vi "CODCr通讯.vi"() -> ()   [LabVIEW 2016, in "CODCr库.lvlib"]
uses:
  <vilib>/Plasmionique/MB Master/MB_Master_TCP/MB_Master_TCP.lvclass
  D:/Program Files (x86)/National Instruments/LabVIEW 2016/vi.lib/Plasmionique/MB Master/MB_Master/MB_Master.lvclass
  <vilib>/NI/Modbus Library/API/Wrapper/Create TCP Slave.vi
  <vilib>/NI/Modbus Library/API/slave/Modbus Slave.lvclass
  <vilib>/Plasmionique/MB Master/MB Master.lvlib
  <vilib>/Utility/config.llb/NI_LVConfig.lvlib
  <vilib>/NI/Modbus Library/API/Wrapper/API Main.lvlib
  <vilib>/Plasmionique/MB Master/MB_Master/MB_Master.lvclass
panel:
  out "状态告警区":u16[](array[numeric])
  out "测量数据区":u16[](array[numeric])
  in  "读取参数":bool
  in  "读取数据":bool
  in  "释放串口":bool
  in  "打开串口":bool
  out "队列中元素数量":i32
  out "元素":cluster{"命令":string}[](array[cluster])
  out "待处理插入数量":i32
  out "读取公式":u16[](array[numeric])
  out "读取参数":u16[](array[numeric])
  out "数据存储":u16[](array[numeric])
  out "通讯状态":bool
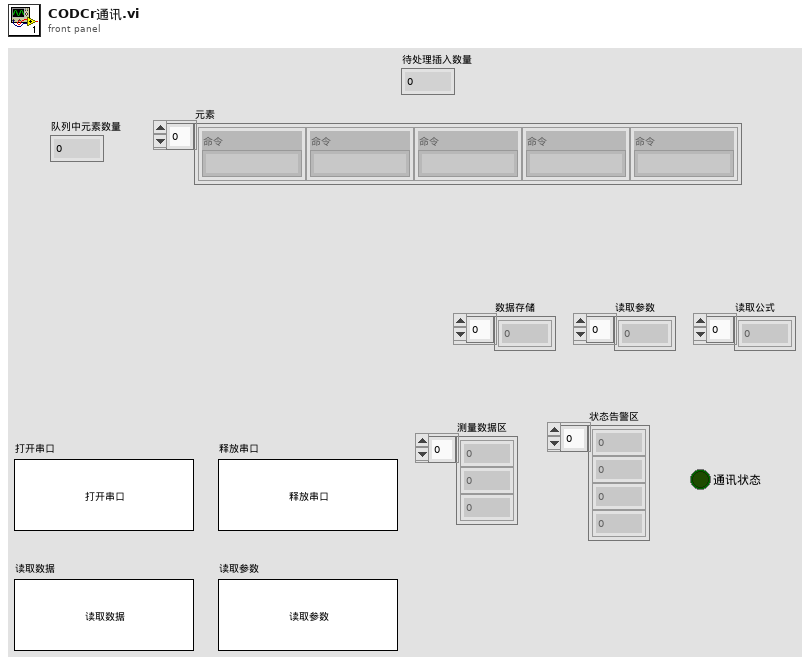
[diagram p1: front panel]
types:
  T1 = typedef "NI_LVConfig.lvlib/Config Data RefNum.ctl" = refnum<k1>
  T2 = cluster{"因子编码":u32, "单位":u16, "标样参考值":sgl, "水样数据时间":timestamp, "水样实测值":sgl, "水样数据标识":string, "标样数据时间":timestamp, "标样实测值":sgl, "标样数据标识":string, "空白数据时间":timestamp, "空白实测值":sgl, "空白数据标识":string, "零点核查数据时间":timestamp, "零点核查实测值":sgl, "零点核查数据标识":string, "跨度核查数据时间":timestamp, "跨度核查实测值":sgl, "跨度核查数据标识":string, "加标回收数据时间":timestamp, "加标回收实测值":sgl, "加标回收数据标识":string, "平行样数据时间":timestamp, "平行样实测值":sgl, "平行样数据标识":string}
  T3 = cluster{"系统时间":timestamp, "工作状态":enum16{"空闲", "水样测试", "标样核查", "零点核查", "跨度核查", "空白测试", "平行样测试", "加标回收", "空白校准", "标样校准", "初始化（清洗）"}, "测量模式":enum16{"待机", "连续模式", "周期模式", "定点模式", "受控模式", "手动模式"}, "告警代码":enum16{"无告警", "缺试剂告警", "缺水样告警", "缺蒸馏水告警", "缺标液告警", "仪表漏液告警", "标定异常告警", "超量程告警", "加热异常", "低试剂预警", "超上限告警", "超下限告警", "仪表内部其他异常", "滴定异常告警", "电极异常告警", "量程切换告警", "参数设置告警", "PH电极电位异常", "电导率电极异常", "浊度光度异常", "溶解氧电极异常", "溶解氧光强异常", "温度异常告警", "PH异常告警", "溶解氧异常告警", "电导率异常告警", "浊度异常告警", "叶绿素异常告警", "藻密度异常告警", "蓝绿藻异常告警", "ORP异常告警", "氨氮异常告警", "清洁刷异常告警", "SD卡异常告警", "蓝牙异常告警", "Wifi异常告警", "流程异常告警"}, "故障代码":enum16{"无故障", "电机故障", "温度故障", "通讯故障", "滴定故障"}, "日志代码":u16, "软件版本":u16, "F0":sgl, "F1":sgl, "F2":sgl, "F3":sgl, "T":sgl, "H":sgl, "id":u16, "flowid":u16, "量程":u16}
  T4 = cluster{"测量精度":u16, "消解温度":u16, "消解时长":u16, "量程下限":sgl, "量程上限":sgl, "曲线斜率K":sgl, "曲线斜率B":sgl, "标定日期":timestamp, "标液1浓度":sgl, "标液1测量过程值":sgl, "标液2浓度":sgl, "标液2测量过程值":sgl, "标液3浓度":sgl, "标液3测量过程值":sgl, "标液4浓度":sgl, "标液4测量过程值":sgl, "标液5浓度":sgl, "标液5测量过程值":sgl, "线性相关系数":sgl, "试剂余量":u32, "测量滴定值或吸光度":sgl, "空白校准时间":timestamp, "标样校准时间":timestamp, "检出限值":sgl, "校准系数":sgl, "设备系列号":string}
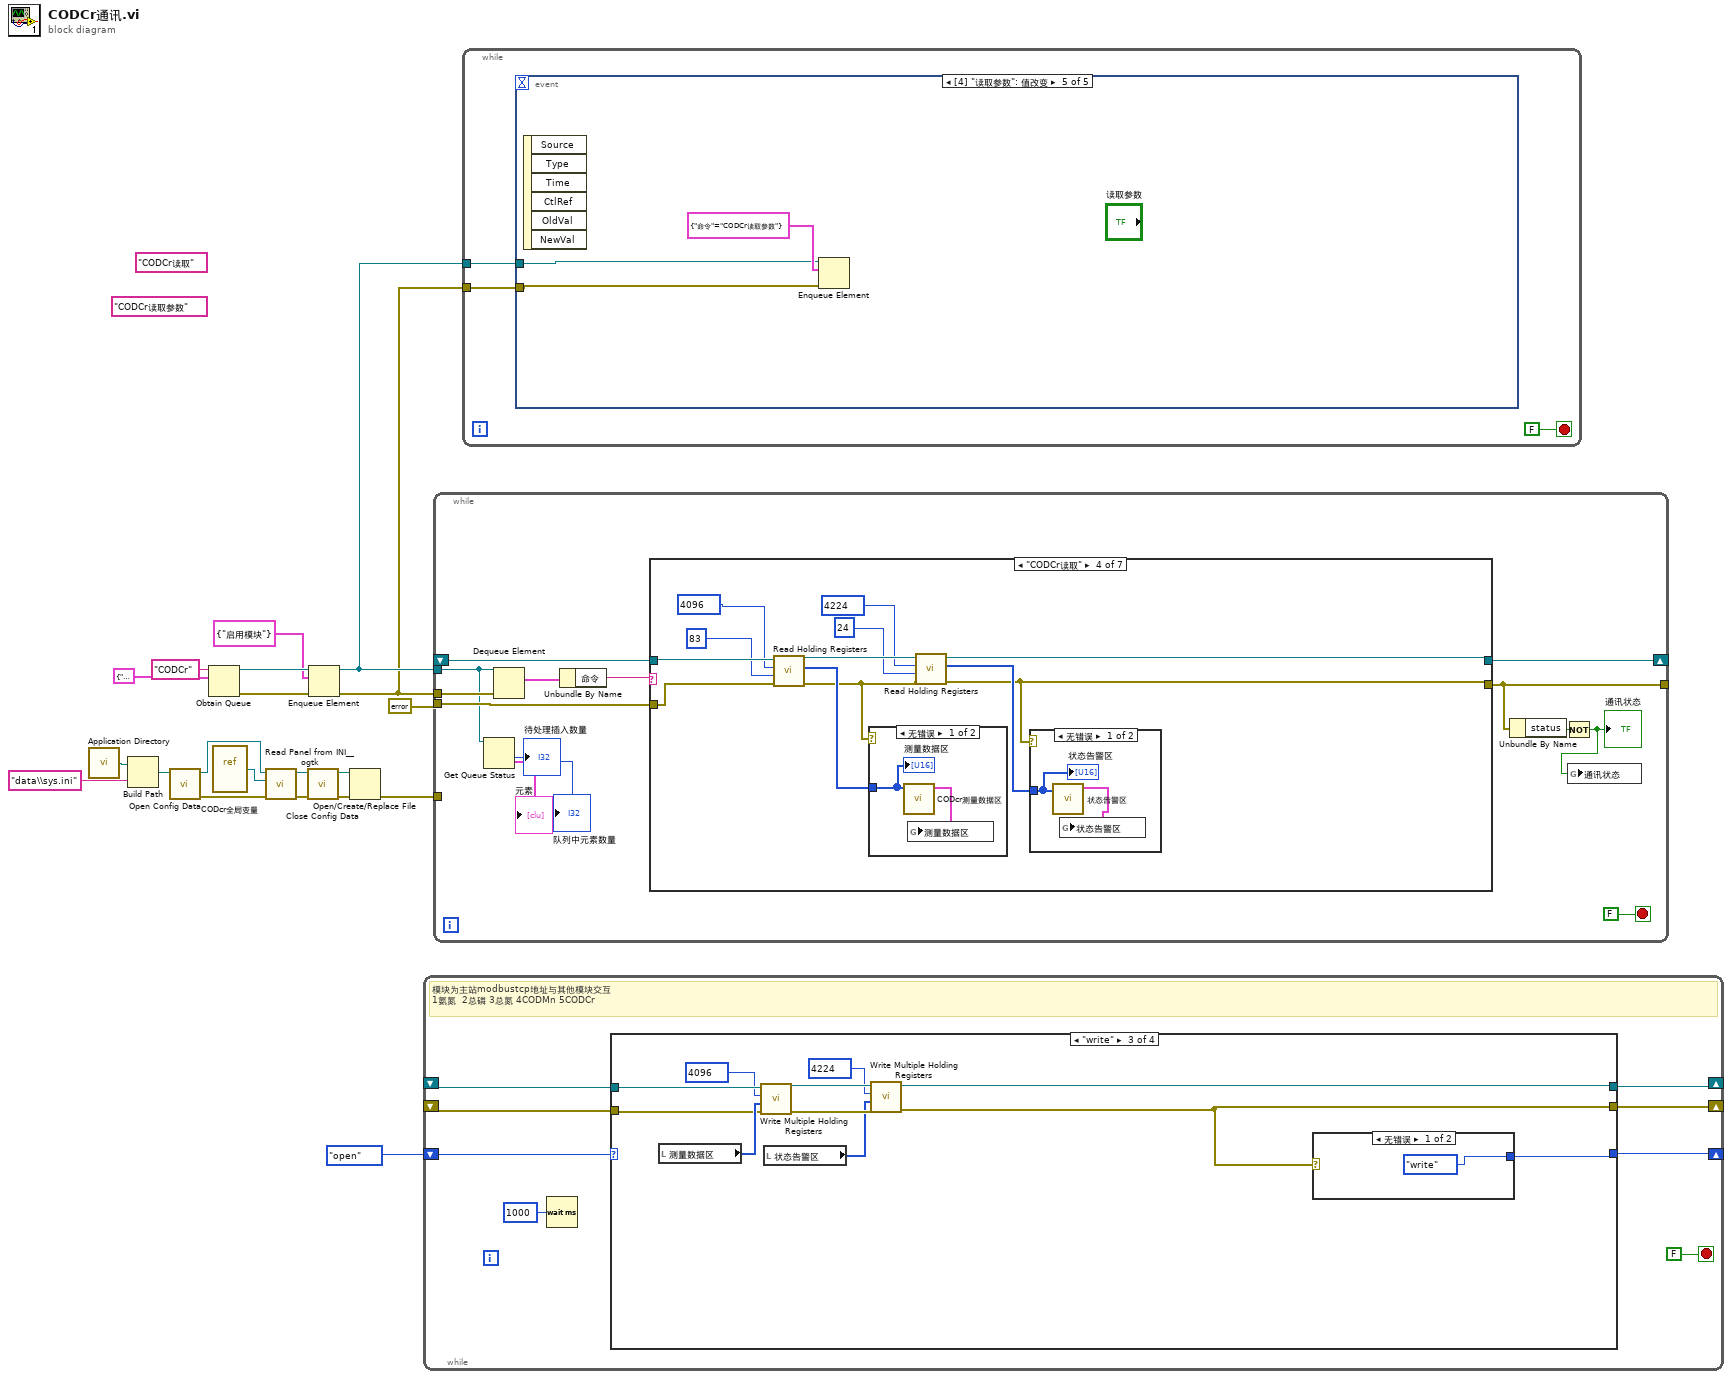
[diagram p0: block diagram]
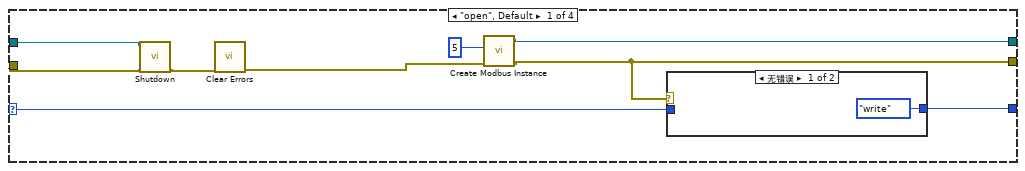
[diagram p2: hidden frame]
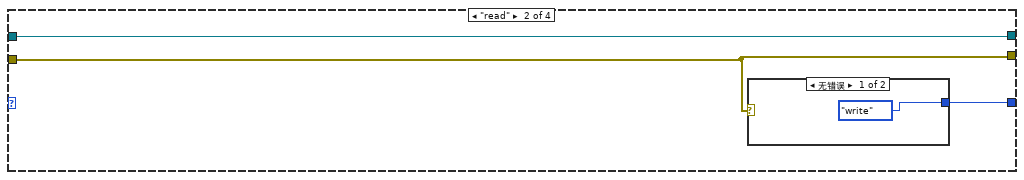
[diagram p4: hidden frame]
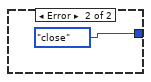
[diagram p5: hidden frame]
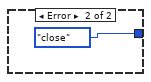
[diagram p6: hidden frame]
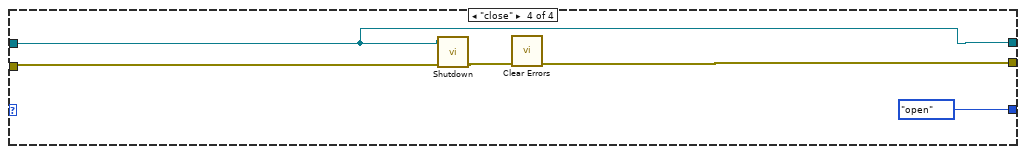
[diagram p7: hidden frame]
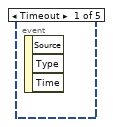
[diagram p8: hidden frame]
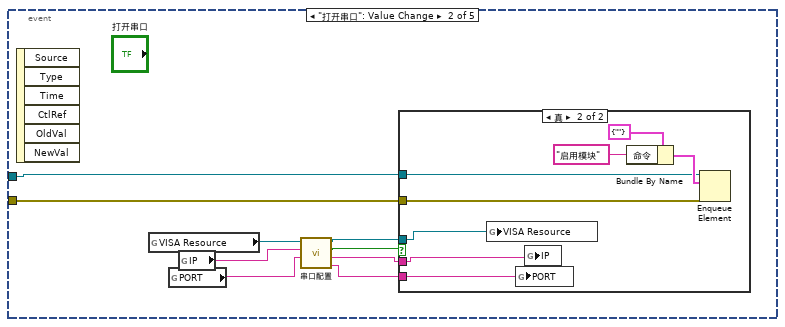
[diagram p9: hidden frame]
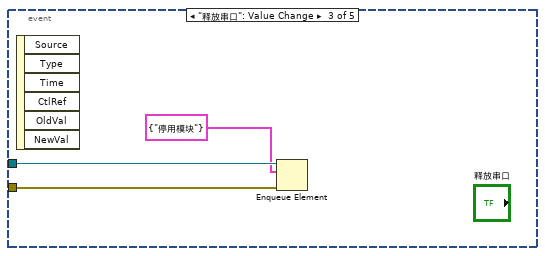
[diagram p11: hidden frame]
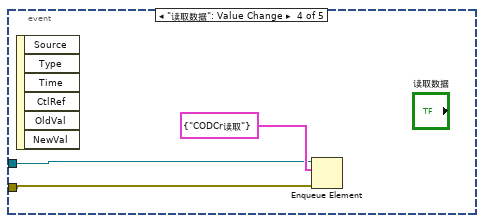
[diagram p12: hidden frame]
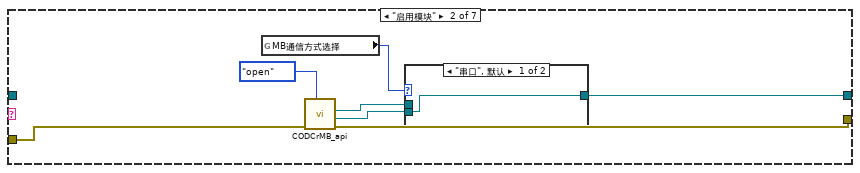
[diagram p14: hidden frame]
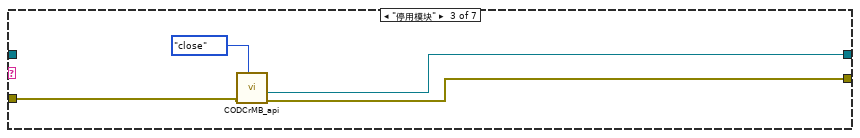
[diagram p16: hidden frame]
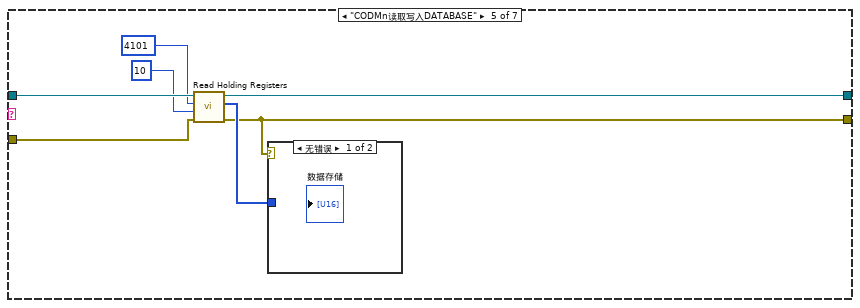
[diagram p19: hidden frame]
diagram:
  (unwired) "CODCr读取参数" ("名称（未命名）")
  (unwired) "CODCr读取" ("名称（未命名）")
  n1 = call <vilib>:"Application Directory.vi"() -> ("Application Directory"=w14:path)
  n2 = Build Path(base path=w14, name or relative path="data\\sys.ini" ("名称或相对路径")) -> (appended path=w12:path)
  n3 = call <vilib>:"Open Config Data.vi"("configuration file path"=w12) -> ("error out"=w8:errorcluster, "refnum"=w11:T1)  [unwired: 8 in, 1 out]
  n4 = Obtain Queue(name (unnamed)="CODCr" ("名称（未命名）"), element data type=cluster{"命令":string} {"命令"="启用模块"} ("元素")) -> (queue out=w17:refnum<queue>, error out=w16:errorcluster)  [unwired: 3 in, 1 out]
  n5 = vi-ref "CODcr全局变量.vi"() -> (w10:refnum<vi>)
  n6 = call <userlib>:"Read Panel from INI__ogtk.vi"("error in (no error)"=w8, "VI ref"=w10, "refnum"=w11) -> ("error out"=w7:errorcluster, "refnum out"=w9:T1)  [unwired: 7 in]
  n7 = call <vilib>:"Close Config Data.vi"("error in (no error)"=w7, "refnum"=w9) -> ("error out"=w6:errorcluster, "file path"=w5:path)  [unwired: 8 in]
  n8 = Enqueue Element(queue=w17, element=cluster{"命令":string} {"命令"="启用模块"} ("元素"), error in (no error)=w16) -> (queue out=w3:refnum<queue>, error out=w2:errorcluster)  [unwired: 1 in, 1 out]
  n9 = Open/Create/Replace File(file path (use dialog)=w5, error in=w6) -> (error out=w4:errorcluster)  [unwired: 4 in, 2 out]
  n10 = while {
    shift-right: [w26] -> _
    shift-left: _ -> [w28]
    shift-right: [w25] -> _
    shift-left: _ -> [w27]
    shift-right: [w22] -> _
    shift-left: enum16{"open", "read", "write", "close"}."open" -> [w23]
    stop <- FALSE stop-if-true
    # "模块为主站modbustcp地址与其他模块交互\n1氨氮  2总磷 3总氮 4CODMn 5CODCr"
    n11 = Wait (ms)(milliseconds to wait=u32 1000 ("等待时间（毫秒）")) -> ()  [unwired: 1 out]
    n12 = case shown="\"write\"" w23 {
      selector: w23 -> [w37 _ _ _]
      tunnel: w28 -> [w31 w40 w54 w60]
      tunnel: w27 -> [w30 w41 w50 w59]
      tunnel: [w34 w40 w46 w60] -> w26
      tunnel: [w33 w41 w45 w62] -> w25
      tunnel: [w36 w42 w55 enum16{"open", "read", "write", "close"}."open"] -> w22
      frame "open", Default {
        n13 = call-dynamic "Shutdown.vi"("error in"=w30, "Modbus slave in"=w31) -> ("error out"=w29:errorcluster)  [unwired: 9 in]
        n14 = call <vilib>:"Clear Errors.vi"("error in (no error)"=w29) -> ("error out"=w32:errorcluster)  [unwired: 5 in, 1 out]
        n15 = call-poly <vilib>:"Create Modbus Instance.vi"("error in"=w32, "port (502)"=u16 5) -> ("error out"=w33:errorcluster, "TCP slave instance"=w34:refnum<class "Modbus Slave.lvclass">)  [unwired: 8 in]
        n16 = case shown="无错误" w33 {
          tunnel: w37 -> [_ w39]
          tunnel: [enum16{"open", "read", "write", "close"}."write" w39] -> w36
          frame No Error {
          }
          frame Error {
          }
        }
      }
      frame "read" {
        n17 = case shown="无错误" w41 {
          tunnel: [enum16{"open", "read", "write", "close"}."write" enum16{"open", "read", "write", "close"}."close"] -> w42
          frame No Error {
          }
          frame Error {
          }
        }
      }
      frame "write" {
        n18 = local read "测量数据区"() -> (w52:u16[])
        n19 = call-dynamic "Write Multiple Holding Registers.vi"("error in"=w50, "registers to write"=w52, "starting address"=u16 4096, "Modbus slave in"=w54) -> ("error out"=w49:errorcluster, "Modbus slave out"=w51:refnum<class "Modbus Slave.lvclass">)  [unwired: 6 in]
        n20 = local read "状态告警区"() -> (w47:u16[])
        n21 = call-dynamic "Write Multiple Holding Registers.vi"("error in"=w49, "registers to write"=w47, "starting address"=u16 4224, "Modbus slave in"=w51) -> ("error out"=w45:errorcluster, "Modbus slave out"=w46:refnum<class "Modbus Slave.lvclass">)  [unwired: 6 in]
        n22 = case shown="无错误" w45 {
          tunnel: [enum16{"open", "read", "write", "close"}."write" enum16{"open", "read", "write", "close"}."close"] -> w55
          frame No Error {
          }
          frame Error {
          }
        }
      }
      frame "close" {
        n23 = call-dynamic "Shutdown.vi"("error in"=w59, "Modbus slave in"=w60) -> ("error out"=w58:errorcluster)  [unwired: 9 in]
        n24 = call <vilib>:"Clear Errors.vi"("error in (no error)"=w58) -> ("error out"=w62:errorcluster)  [unwired: 5 in, 1 out]
      }
    }
  }
  n25 = while {
    tunnel: w3 -> [w66]
    tunnel: w2 -> [w75]
    tunnel: [w67] -> _
    shift-right: [w71] -> _
    shift-left: _ -> [w70]
    tunnel: errorcluster {"status"=FALSE, "code"=0, "source"=""} ("error out") -> [w69]
    tunnel: w4 -> [_]
    stop <- FALSE stop-if-true
    n26 = Get Queue Status(queue=w66) -> (# pending insert=→"待处理插入数量":i32, # elements in queue=→"队列中元素数量":i32, elements=→"元素":cluster{"命令":string}[])  [unwired: 2 in, 5 out]
    n27 = Dequeue Element(queue=w66, error in (no error)=w75) -> (element=w74:cluster{"命令":string})  [unwired: 1 in, 3 out]
    n28 = Unbundle By Name(w74) -> ("命令"=w73:string)
    n29 = case shown="\"CODCr读取\"" w73 {
      tunnel: [w78 w79 w88 w97 w110 w118 w127] -> w71
      tunnel: [w77 w85 w89 w96 w108 w117 w126] -> w67
      tunnel: w70 -> [w78 _ _ w103 w114 w121 w130]
      tunnel: w69 -> [w77 w83 w90 w102 w111 w120 w129]
      frame Default {
      }
      frame "启用模块" {
        n30 = global read "CODcr全局变量.vi" "MB通信方式选择"() -> (w82:enum16{"串口", "TCP"})
        n31 = call "CODCrMB_api.vi"("STEP"=enum16{"open", "read", "write", "close"}."open", "Error in"=w83) -> ("error out"=w85:errorcluster, "MB session out"=w81:refnum<class "MB_Master.lvclass">, "MB_TCP session"=w80:refnum<class "MB_Master_TCP.lvclass">)  [unwired: 6 in, 1 out]
        n32 = case shown="\"串口\", 默认" w82 {
          tunnel: w81 -> [w86 _]
          tunnel: w80 -> [_ w87]
          tunnel: [w86 w87] -> w79
          frame "串口", Default {
          }
          frame "TCP" {
          }
        }
      }
      frame "停用模块" {
        n33 = call "CODCrMB_api.vi"("STEP"=enum16{"open", "read", "write", "close"}."close", "Error in"=w90) -> ("error out"=w89:errorcluster, "MB session out"=w88:refnum<class "MB_Master.lvclass">)  [unwired: 6 in, 2 out]
      }
      frame "CODCr读取" {
        n34 = call <vilib>:"Read Holding Registers.vi"("error in (no error)"=w102, "quantity"=u16 83 ("number of holding registers"), "starting address"=u16 4096, "MB session in"=w103) -> ("error out"=w99:errorcluster, "Registers"=w101:u16[], "MB session out"=w100:refnum<class "MB_Master.lvclass">)  [unwired: 5 in]
        n35 = case shown="无错误" w99 {
          tunnel: w101 -> [w106 _]
          frame No Error {
            n36 = call "CODcr测量数据区.vi"("数组"=w106) -> ("测量数据区"=w107:T2)  [unwired: 10 in]
            n37 = global write "CODcr全局变量.vi" "测量数据区"(w107) -> ()
            "测量数据区" <- w106
          }
          frame Error {
          }
        }
        n38 = call <vilib>:"Read Holding Registers.vi"("error in (no error)"=w99, "quantity"=u16 24 ("number of holding registers"), "starting address"=u16 4224, "MB session in"=w100) -> ("error out"=w96:errorcluster, "Registers"=w98:u16[], "MB session out"=w97:refnum<class "MB_Master.lvclass">)  [unwired: 5 in]
        n39 = case shown="无错误" w96 {
          tunnel: w98 -> [w104 _]
          frame No Error {
            n40 = call "状态告警区.vi"("数组"=w104) -> ("状态告警区"=w105:T3)  [unwired: 10 in]
            n41 = global write "CODcr全局变量.vi" "状态告警区"(w105) -> ()
            "状态告警区" <- w104
          }
          frame Error {
          }
        }
      }
      frame "CODMn读取写入DATABASE" {
        n42 = call <vilib>:"Read Holding Registers.vi"("error in (no error)"=w111, "quantity"=u16 10 ("number of holding registers"), "starting address"=u16 4101, "MB session in"=w114) -> ("error out"=w108:errorcluster, "Registers"=w109:u16[], "MB session out"=w110:refnum<class "MB_Master.lvclass">)  [unwired: 5 in]
        n43 = case shown="无错误" w108 {
          tunnel: w109 -> [_ _]
          frame No Error {
          }
          frame Error {
          }
        }
      }
      frame "CODCr读取参数" {
        n44 = call <vilib>:"Read Holding Registers.vi"("error in (no error)"=w120, "quantity"=u16 19 ("number of holding registers"), "starting address"=u16 4256, "MB session in"=w121) -> ("error out"=w117:errorcluster, "Registers"=w119:u16[], "MB session out"=w118:refnum<class "MB_Master.lvclass">)  [unwired: 5 in]
        n45 = case shown="无错误" w117 {
          tunnel: w119 -> [w122 _]
          frame No Error {
            n46 = call "关键参数区.vi"("数组"=w122) -> ("关键参数区"=w123:T4)  [unwired: 10 in]
            n47 = global write "CODcr全局变量.vi" "关键参数区"(w123) -> ()
          }
          frame Error {
          }
        }
      }
      frame "CODMn读取公式" {
        n48 = call <vilib>:"Read Holding Registers.vi"("error in (no error)"=w129, "quantity"=u16 94 ("number of holding registers"), "starting address"=u16 4616, "MB session in"=w130) -> ("error out"=w126:errorcluster, "Registers"=w128:u16[], "MB session out"=w127:refnum<class "MB_Master.lvclass">)  [unwired: 5 in]
        n49 = case shown="无错误" w126 {
          tunnel: w128 -> [_ _]
          frame No Error {
          }
          frame Error {
          }
        }
      }
    }
    n50 = Unbundle By Name(w67) -> ("status"=w72:bool)
    n51 = Not(x=w72) -> (.not. x?=w68:bool)
    "通讯状态" <- w68
    n52 = global write "CODcr全局变量.vi" "通讯状态"(w68) -> ()
  }
  n53 = while {
    tunnel: w3 -> [w132]
    tunnel: w2 -> [w131]
    stop <- FALSE stop-if-true
    n54 = event shown="[4] \"读取参数\": 值改变" {
      selector: _ -> [_ _ _ _ _]
      dyn-events: _ -> [_ _ _ _ _]
      timeout: _ -> [_ _ _ _ _]
      tunnel: w132 -> [_ w142 w153 w155 w158]
      tunnel: w131 -> [_ w141 w152 w154 w157]
      event Timeout {
        n55 = event-data() -> ()  [unwired: 1 in, 3 out]
      }
      event "打开串口": Value Change {
        n56 = event-data() -> ()  [unwired: 1 in, 6 out]
        n57 = global read "CODcr全局变量.vi" "VISA Resource"() -> (w140:refnum<visa-resource-name>)
        n58 = global read "CODcr全局变量.vi" "PORT"() -> (w134:string)
        n59 = global read "CODcr全局变量.vi" "IP"() -> (w135:string)
        n60 = call "串口配置.vi"("PORT"=w134, "IP"=w135, "请选择串口:"=w140) -> ("PORT 2"=w136:string, "IP 2"=w137:string, "确认 2"=w139:bool, "VISA资源名称 2"=w138:refnum<visa-resource-name>)  [unwired: 5 in]
        n61 = case shown="真" w139 {
          tunnel: w138 -> [_ w145]
          tunnel: w142 -> [_ w147]
          tunnel: w141 -> [_ w146]
          tunnel: w137 -> [_ w144]
          tunnel: w136 -> [_ w143]
          frame False {
          }
          frame True {
            n62 = global write "CODcr全局变量.vi" "VISA Resource"(w145) -> ()
            n63 = global write "CODcr全局变量.vi" "PORT"(w143) -> ()
            n64 = global write "CODcr全局变量.vi" "IP"(w144) -> ()
            n65 = Bundle By Name(cluster=cluster{"命令":string} {"命令"=""} ("元素"), "命令"="启用模块" ("名称（未命名）")) -> (w148:cluster{"命令":string})
            n66 = Enqueue Element(queue=w147, element=w148, error in (no error)=w146) -> ()  [unwired: 1 in, 3 out]
          }
        }
      }
      event "释放串口": Value Change {
        n67 = event-data() -> ()  [unwired: 1 in, 6 out]
        n68 = Enqueue Element(queue=w153, element=cluster{"命令":string} {"命令"="停用模块"} ("元素"), error in (no error)=w152) -> ()  [unwired: 1 in, 3 out]
      }
      event "读取数据": Value Change {
        n69 = event-data() -> ()  [unwired: 1 in, 6 out]
        n70 = Enqueue Element(queue=w155, element=cluster{"命令":string} {"命令"="CODCr读取"} ("元素"), error in (no error)=w154) -> ()  [unwired: 1 in, 3 out]
      }
      event "读取参数": Value Change {
        n71 = event-data() -> ()  [unwired: 1 in, 6 out]
        n72 = Enqueue Element(queue=w158, element=cluster{"命令":string} {"命令"="CODCr读取参数"} ("元素"), error in (no error)=w157) -> ()  [unwired: 1 in, 3 out]
      }
    }
  }
